vi "SeCrTs-RT Connected .vi"(7 "Enum":enum16{"Read", "Write"}(ring), 8 "error in":errorcluster, 10 "Pumb rt con":bool, 11 "Storage rt con":bool) -> (0 "error out":errorcluster, 2 "Pumb rt con R":bool, 3 "Stoarge rt con R":bool)   [LabVIEW 2022 SP3]
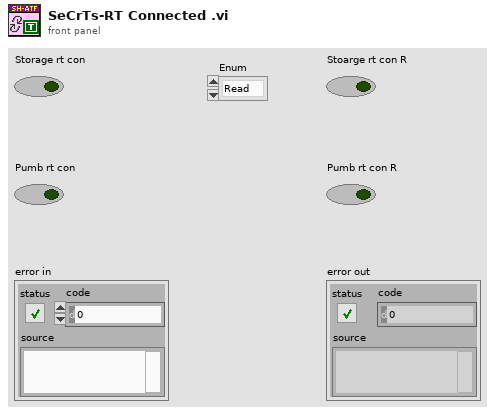
[diagram p1: front panel]
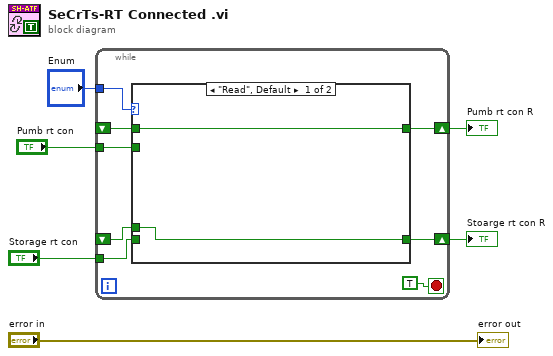
[diagram p0: block diagram]
diagram:
  n1 = while {
    tunnel: "Enum" -> [w14]
    tunnel: "Storage rt con" -> [w12]
    shift-right: [w11] -> w3
    shift-left: _ -> [w10]
    tunnel: "Pumb rt con" -> [w8]
    shift-right: [w9] -> w2
    shift-left: _ -> [w7]
    stop <- TRUE stop-if-true
    n2 = case shown="\"Read\", Default" w14 {
      tunnel: w12 -> [_ w18]
      tunnel: [w16 w18] -> w11
      tunnel: w10 -> [w16 _]
      tunnel: [w15 w17] -> w9
      tunnel: w8 -> [_ w17]
      tunnel: w7 -> [w15 _]
      frame "Read", Default {
      }
      frame "Write" {
      }
    }
  }
  "Stoarge rt con R" <- w3
  "Pumb rt con R" <- w2
  "error out" <- "error in"
